vi "I2C LCD - Print String Array.vi"(7 "Back Light":bool, 8 "error in (no error)":errorcluster, 9 "Slave Address (7-bit)":u8, 10 "String Array":string[](array[string]), 11 "I2C Ref  in":T1) -> (0 "error out":errorcluster, 3 "I2C Ref Out":T1)   [LabVIEW 2017]
uses:
  <vilib>/myRIO/Instrument Drivers/Onboard IO/I2C/typedefs/I2C Reference.ctl
  <vilib>/myRIO/Common/Instrument Driver Framework/Utilities/typedefs/myRIO Generic Hardware Reference.ctl
  <vilib>/myRIO/Common/Instrument Driver Framework/Utilities/typedefs/Hardware Version Enum.ctl
  <vilib>/myRIO/Common/Instrument Driver Framework/Utilities/typedefs/myRIO v1.0 Reference.ctl
  <vilib>/myRIO/Common/Instrument Driver Framework/Utilities/typedefs/Generic FPGA Reference.ctl
  <vilib>/myRIO/Common/Instrument Driver Framework/myRIO v1.0/I2C/typedefs/I2C Channels Enum.ctl
  <vilib>/myRIO/Instrument Drivers/Onboard IO/I2C/typedefs/I2C Configuration.ctl
  <vilib>/myRIO/Instrument Drivers/Onboard IO/I2C/typedefs/I2C Transfer Rate.ctl
  <vilib>/myRIO/Instrument Drivers/Onboard IO/I2C/I2C.lvlib
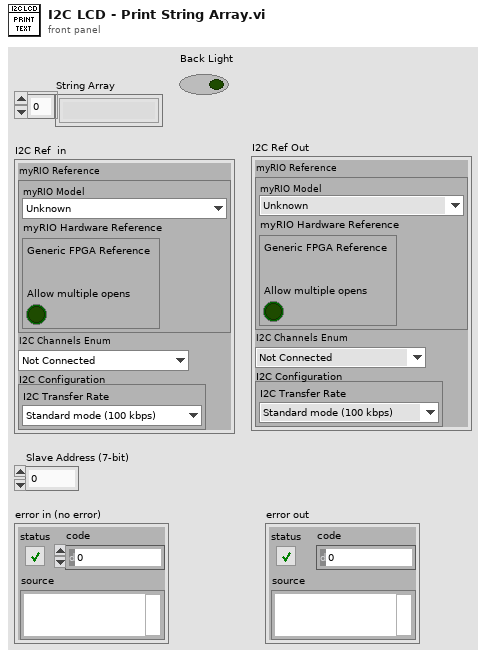
[diagram p1: front panel]
types:
  T1 = typedef "I2C.lvlib/I2C Reference.ctl" = cluster{"myRIO Reference":T2, "I2C Channels Enum":T6, "I2C Configuration":T7}
  T2 = typedef "myRIO Generic Hardware Reference.ctl" = cluster{"myRIO Model":T3, "myRIO Hardware Reference":T4}
  T3 = typedef "Hardware Version Enum.ctl" = enum16{"Unknown", "myRIO-1900", "myRIO-1950", "roboRIO", "NI ELVIS RIO CM"}
  T4 = typedef "myRIO v1.0 Reference.ctl" = cluster{"Generic FPGA Reference":T5, "Allow multiple opens":bool}
  T5 = typedef "Generic FPGA Reference.ctl" = refnum<k20>
  T6 = typedef "I2C Channels Enum.ctl" = enum16{"Not Connected", "A/I2C", "B/I2C", "I2C/I2C"}
  T7 = typedef "I2C.lvlib/I2C Configuration.ctl" = cluster{"I2C Transfer Rate":T8}
  T8 = typedef "I2C.lvlib/I2C Transfer Rate.ctl" = enum16{"Standard mode (100 kbps)", "Fast mode (400 kbps)"}
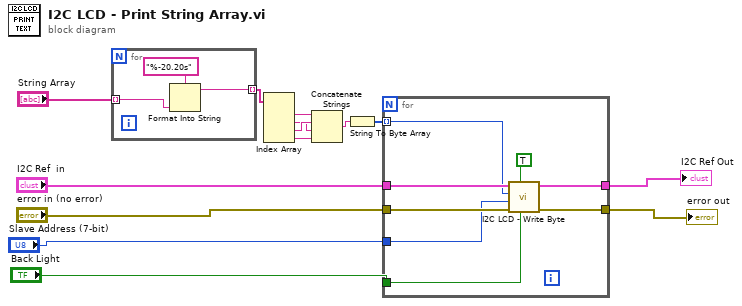
[diagram p0: block diagram]
diagram:
  n1 = for {
    tunnel: "String Array" -> [w17] mode=indexing
    tunnel: [w15] -> w7 mode=indexing
    n2 = Format Into String(format string="%-20.20s", w17) -> (resulting string=w15:string)  [unwired: 2 in, 1 out]
  }
  n3 = Index Array(array=w7) -> (element #1=w8:string, element #2=w9:string, element #3=w10:string, element #4=w11:string)  [unwired: 4 in]
  n4 = Concatenate Strings(w8, w10, w9, w11) -> (w12:string)
  n5 = String To Byte Array(string=w12) -> (unsigned byte array=w5:u8[])
  n6 = for {
    tunnel: "error in (no error)" -> [w23]
    tunnel: "I2C Ref  in" -> [w24]
    tunnel: "Slave Address (7-bit)" -> [w20]
    tunnel: [w25] -> w13
    tunnel: [w22] -> w14
    tunnel: w5 -> [w21] mode=indexing
    tunnel: "Back Light" -> [w19]
    n7 = call "I2C LCD - Write Byte.vi"("BL"=w19, "RS"=TRUE, "error in (no error)"=w23, "Slave Address (7-bit)"=w20, "Numeric"=w21, "I2C Ref"=w24) -> ("error out"=w22:errorcluster, "I2C Ref Out"=w25:T1)  [unwired: 4 in]
  }
  "error out" <- w14
  "I2C Ref Out" <- w13
